vi "readEtherneModeFromXml.vi"(6 "type":string, 8 "error in (no error)":errorcluster, 9 "device.lvclass":refnum<class "device.lvclass">, 10 "xml in":refnum<class "NativeXML.lvclass">, 11 "deviceDataBase in":refnum<class "deviceDataBase.lvclass">) -> (0 "error out":errorcluster, 1 "device.lvclass out":refnum<class "device.lvclass">, 2 "xml out":refnum<class "NativeXML.lvclass">, 3 "deviceDataBase out":refnum<class "deviceDataBase.lvclass">)   [LabVIEW 2011, in "Tools.lvlib" / "DatabaseHelpers.lvlib" / "deviceDataBase.lvclass"]
uses:
  deviceDataBase.lvclass
  Database Objects/device/device.lvclass
  NativeXML/NativeXML.lvclass
  Database Objects/device/EthernetSupply/ethernetSupply.lvclass
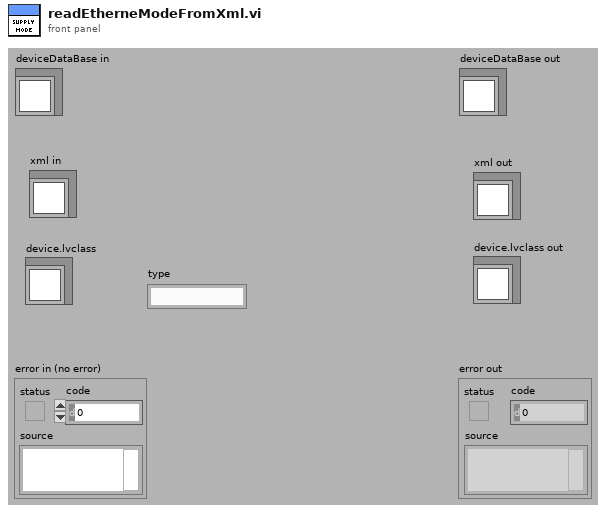
[diagram p1: front panel]
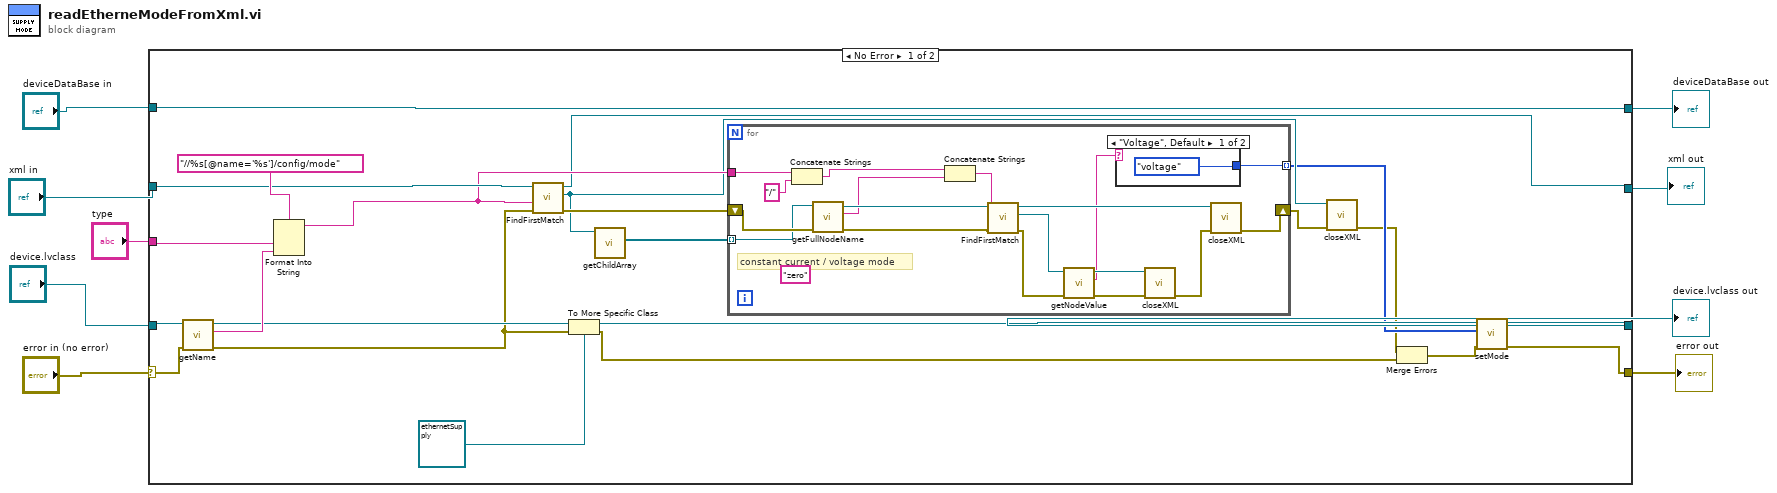
[diagram p0: block diagram]
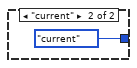
[diagram p2: hidden frame]
diagram:
  n1 = case shown="No Error" "error in (no error)" {
    selector: "error in (no error)" -> [w30 w56]
    tunnel: [w10 w56] -> w7
    tunnel: [w32 w55] -> w8
    tunnel: "xml in" -> [w26 w54]
    tunnel: "device.lvclass" -> [w31 w53]
    tunnel: [w11 w53] -> w2
    tunnel: [w24 w54] -> w3
    tunnel: "deviceDataBase in" -> [w32 w55]
    tunnel: "type" -> [w29 _]
    frame No Error {
      n2 = call "getName.vi"("error in (no error)"=w30, "device.lvclass in"=w31) -> ("error out"=w21:errorcluster, "name"=w28:string, "device.lvclass out"=w22:refnum<class "device.lvclass">)  [unwired: 7 in]
      n3 = Format Into String(format string="//%s[@name='%s']/config/mode", w29, w28) -> (resulting string=w25:string)  [unwired: 2 in, 1 out]
      n4 = call "FindFirstMatch.vi"("error in (no error)"=w21, "xPath"=w25, "NativeXML in"=w26) -> ("error out"=w23:errorcluster, "NativeXML match"=w17:refnum<class "NativeXML.lvclass">, "NativeXML out"=w24:refnum<class "NativeXML.lvclass">)  [unwired: 6 in]
      n5 = To More Specific Class(target class=refnum<class "ethernetSupply.lvclass"> refnum ("Tools.lvlib:DatabaseHelpers.lvlib:ethernetSupply.lvclass"), reference=w22, error in=w21) -> (specific class reference=w19:refnum<class "ethernetSupply.lvclass">, error out=w12:errorcluster)
      n6 = call "getChildArray.vi"("NativeXML in"=w17) -> ("childArray"=w18:refnum<class "NativeXML.lvclass">[])  [unwired: 8 in, 2 out]
      n7 = for {
        tunnel: w25 -> [w49]
        tunnel: w18 -> [w38] mode=indexing
        shift-right: [w35] -> w16
        shift-left: w23 -> [w42]
        tunnel: [w33] -> w15 mode=indexing
        (unwired) "zero"
        # "constant current / voltage mode"
        n8 = Concatenate Strings(w49, "/") -> (w41:string)
        n9 = call "getFullNodeName.vi"("error in (no error)"=w42, "NativeXML in"=w38) -> ("error out"=w39:errorcluster, "fullName"=w40:string, "NativeXML out"=w46:refnum<class "NativeXML.lvclass">)  [unwired: 7 in]
        n10 = Concatenate Strings(w41, w40) -> (w43:string)
        n11 = call "FindFirstMatch.vi"("error in (no error)"=w39, "xPath"=w43, "NativeXML in"=w46) -> ("error out"=w45:errorcluster, "NativeXML match"=w44:refnum<class "NativeXML.lvclass">, "NativeXML out"=w37:refnum<class "NativeXML.lvclass">)  [unwired: 6 in]
        n12 = call "getNodeValue.vi"("error in (no error)"=w45, "NativeXML in"=w44) -> ("error out"=w47:errorcluster, "Value"=w34:string, "NativeXML out"=w48:refnum<class "NativeXML.lvclass">)  [unwired: 7 in]
        n13 = case shown="\"Voltage\", Default" w34 {
          tunnel: [enum16{"current", "voltage"}."voltage" ("mode") enum16{"current", "voltage"}."current" ("mode")] -> w33
          frame "Voltage", Default {
          }
          frame "current" {
          }
        }
        n14 = call "closeXML.vi"("error in (no error)"=w47, "NativeXML in"=w48) -> ("error out"=w36:errorcluster)  [unwired: 9 in]
        n15 = call "closeXML.vi"("error in (no error)"=w36, "NativeXML in"=w37) -> ("error out"=w35:errorcluster)  [unwired: 9 in]
      }
      n16 = call "closeXML.vi"("error in (no error)"=w16, "NativeXML in"=w17) -> ("error out"=w14:errorcluster)  [unwired: 9 in]
      n17 = Merge Errors(w14, w12) -> (w13:errorcluster)
      n18 = call "setMode.vi"("error in (no error)"=w13, "mode"=w15, "ethernetSupply in"=w19) -> ("error out"=w10:errorcluster, "ethernetSupply out"=w11:refnum<class "ethernetSupply.lvclass">)  [unwired: 7 in]
    }
    frame Error {
    }
  }
  "error out" <- w7
  "deviceDataBase out" <- w8
  "xml out" <- w3
  "device.lvclass out" <- w2
